vi "Alle Frontpanels auslesen.vi"(8 "Fehler (Eingang, kein Fehler)":errorcluster) -> (0 "Fehler (Ausgang)":errorcluster)   [LabVIEW 2020, in "Sprachverwaltung.lvlib"]
uses:
  Sprachverwaltung.lvlib
  Seiten/System Einstellungen V2/Aktioen FGV System Konstanten.ctl
  VI Anlagengrenzwerte.vi
  VI Gaszuordnung.vi
  VisBx Anzeige.vi
  Seiten/Grafik/VI Graph.vi
  Seiten/Grafik/Einstellungen Diagramme.vi
  VI Konfig FT-IR.vi
  Seiten/FT-IR/Gasliste vergleichen.vi
  Seiten/FT-IR/Algebraic Modul/VI Algebraic Konfig.vi
  Seiten/FT-IR/Get Spectra/get Spectra.vi
  VI Erw. Konfig.vi
  AK-Schnittstelle/Konfig AK.vi
  Seiten/Erweiterte Konfig/Status Steuerung.vi
  Seiten/Erweiterte Konfig/PID-Parameter Druckregler einstellen v2.vi
  Seiten/Erweiterte Konfig/Dichtheitstest.vi
  T90/T90 konfig.vi
  T90/T90 main.vi
  Seiten/FT-IR/Hintergrund durchfuehren.vi
  Seiten/System Einstellungen V2/System und Gaseinstellung V2.vi
  Seiten/Statusuebersicht/VI Statusuebersicht.vi
  Passwortverwaltung/VI Passwortverwaltung.vi
  Passwortverwaltung/Passwortlevel aendern.vi
  VI Anlagengrenzwerte PNS.vi
  PNS/Diagnose PNS.vi
  Allgemein/Runtime beenden.vi
  Allgemein/Bitte Warten.vi
  VI Stoermeldungen.vi
  VI Stoermeldepuffer.vi
  VI Stoermeldung Konfig.vi
  cRIO Ueberwachung/VI Fehlerliste.vi
  Seiten/Grafik/Kurven anzeigen.vi
  EPA 1065/Dichtheitstest 1065-345/Konfig Leak Check.vi
  Seiten/FT-IR/Konfig Recipes.vi
  Seiten/FT-IR/TOOLweb Interface Library/TOOLweb Rezept wechseln.vi
  Allgemein/Diagnose Zykluszeit.vi
  Linearisierung V2/SpanEinstellungen/show LIN Load Errors.vi
  EPA 1065/Interference verificaton 1065-366/Hilfe.vi
  EPA 1065/Interference verificaton 1065-375/VI Interference Konfig.vi
  Seiten/FT-IR/Span/Kalibrierung laden.vi
  VI Konfiguration Kalibriergase.vi
  EPA 1065/Interference verificaton 1065-366/VI Interference Konfig.vi
  Seiten/Erweiterte Konfig/Parameter Druck Sensoren.vi
  Seiten/EL3000/PMA/VI PMA Konfig.vi
  Seiten/EL3000/Allgemeine VI/Kalibrierdaten.vi
  Seiten/EL3000/FID/VI FID Konfig.vi
  Seiten/EL3000/Allgemeine VI/FID Manuell Kalibrieren.vi
  Seiten/EL3000/PMA/Kalibrieren/PMA Manuell Kalibrieren.vi
  Allgemein/SPRACHE.vi
  SysLog/VI SysLog History.vi
  SysLog/SysLog Status.vi
  Seiten/Erweiterte Konfig/Konfig CG-Check/CG-Test.vi
  Seiten/Erweiterte Konfig/Konfig CG-Check/VI CG-Check Konfig.vi
  Linearisierung V2/Gasteiler/Horiba/GDC Manuell.vi
  Backup mit WebDAV/Backup.vi
  Seiten/FT-IR/Span/VI Span Seite.vi
  Seiten/CalGas Aufschaltung/Aufschaltung_Popup.vi
  Auto Kalibrieren/VI Auto Kalibrieren.vi
  Linearisierung V2/VI Linearisierung v2.vi
  O2 Dichtheitstest/O2 main.vi
  Seiten/Erweiterte Konfig/Konfig CG-Check/CG_Auswertung.vi
  Linearisierung V2/Gasteiler/Gasteiler Korrektur.vi
  SprachEditor.vi
  EPA 1065/T90 1065-308/T90 Test Konfig.vi
  Schedule Modul/VI Schedule Seite.vi
  Linearisierung V2/Hintergrund durchfuehren FT-IR.vi
  EPA 1065/Gas Analyzer Drift 1065-550/Drift Verification Konfig.vi
  EPA 1065/HovaCAL Interference verification/VI Interference Konfig.vi
  Seiten/System Einstellungen V2/System Einstellungen V2.lvlib
  Seiten/Anlagengrenzwerte/Anlagengrenzwerte.lvlib
  Seiten/Gaszuordnung AO/Gaszuordnung AO.lvlib
  Seiten/Anlagenuebersicht/VisBx Anzeige/Anlagenuebersicht.lvlib
  Seiten/Grafik/Grafik.lvlib
  Seiten/FT-IR/FT-IR.lvlib
  Seiten/FT-IR/Algebraic Modul/Algebraic Modul.lvlib
  Seiten/FT-IR/Get Spectra/Get Spectra.lvlib
  Seiten/Erweiterte Konfig/Erweiterte Konfig.lvlib
  AK-Schnittstelle/AK-Schnittstelle.lvlib
  T90/T90.lvlib
  Seiten/Statusuebersicht/Statusuebersicht.lvlib
  Passwortverwaltung/Passwort.lvlib
  PNS/PNS.lvlib
  Allgemein/allgemeine Sub-VIs.lvlib
  Stoerungen/Stoerungen.lvlib
  cRIO Ueberwachung/cRIO Ueberwachung.lvlib
  EPA 1065/Dichtheitstest 1065-345/Dichtheitstest 1065-345.lvlib
  Seiten/FT-IR/TOOLweb Interface Library/TOOLweb Interface.lvlib
  Seiten/CalGas Aufschaltung/CalGas Aufschaltung.lvlib
  EPA 1065/Interference verificaton 1065-366/Interference verificaton 1065-366.lvlib
  Seiten/EL3000/PMA/PMA.lvlib
  Seiten/EL3000/FID/FID.lvlib
  Seiten/EL3000/Allgemeine VI/Allgemeine VI.lvlib
  Seiten/EL3000/PMA/Kalibrieren/Kalibrieren.lvlib
  SysLog/SysLog.lvlib
  Backup mit WebDAV/Backup.lvlib
  Seiten/FT-IR/Span/Spanfaktor.lvlib
  Seiten/Erweiterte Konfig/Konfig CG-Check/CG-Check Konfig.lvlib
  Auto Kalibrieren/Auto Kalibrieren.lvlib
  Linearisierung V2/Linearisierung v2.lvlib
  O2 Dichtheitstest/O2 Dichtheitstest.lvlib
  Linearisierung V2/Gasteiler/Horiba/Horiba GDC.lvlib
  Linearisierung V2/Gasteiler/Gasteiler.lvlib
  EPA 1065/T90 1065-308/T90 Test 1065-308.lvlib
  EPA 1065/ANR Test 1065-305/ARN Test 1065-305.lvlib
  EPA 1065/Interference verificaton 1065-375/Interference verificaton 1065-375.lvlib
  Schedule Modul/Schedule Modul.lvlib
  Seiten/Log Konfig/LogKonfig.lvlib
  EPA 1065/Gas Analyzer Drift 1065-550/Gas Analyzer Drift 1065-550.lvlib
  EPA 1065/Interference verificaton 1065-375/PDF_Interface_PDF Protokoll EPA1065_InterferenceVerification.vi
  EPA 1065/Interference verificaton 1065-366/PDF_Interface_PDF Protokoll EPA1065_InterferenceVerification.vi
  EPA 1065/ANR Test 1065-305/PDF_Interface_PDF Protokoll EPA1065_305 ARN.vi
  Linearisierung V2/Protokoll/PDF_Interface_PDF Protokoll EPA1065_307.vi
  Linearisierung V2/Protokoll/Protokoll.lvlib
  Linearisierung V2/Protokoll/PDF_Interface_PDF Protokoll Linearisierung.vi
  Seiten/Erweiterte Konfig/PDF_Interface_PDF Protokoll Dichtheitstest.vi
  O2 Dichtheitstest/PDF_Interface_PDF Protokoll O2 Leaktest.vi
  Hangup Check/PDF_Interface_PDF Protokoll HangUp.vi
  Hangup Check/Hangup Check.lvlib
  T90/PDF_Interface_PDF Protokoll T90.vi
  EPA 1065/T90 1065-308/PDF_Interface_PDF Protokoll EPA1065_308 T90.vi
  EPA 1065/Gas Analyzer Drift 1065-550/PDF_Interface_PDF Protokoll EPA1065_550 Drift.vi
  Linearisierung V2/SpanEinstellungen/SpanEinstellungen.lvlib
  EPA 1065/HovaCAL Interference verification/HovaCAL Interference verificaton.lvlib
panel:
  # "Durch ausführen des VI´s werden alle Frontpanels\ndie man vorher hinzufügt ausgelesen"
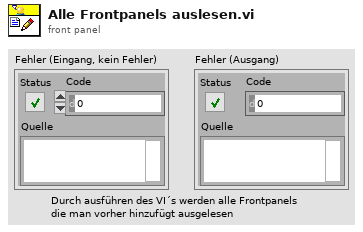
[diagram p1: front panel]
types:
  T1 = typedef "System Einstellungen V2.lvlib/Aktioen FGV System Konstanten.ctl" = enum16{"lesen", "laden", "speichern", "Sprache"}
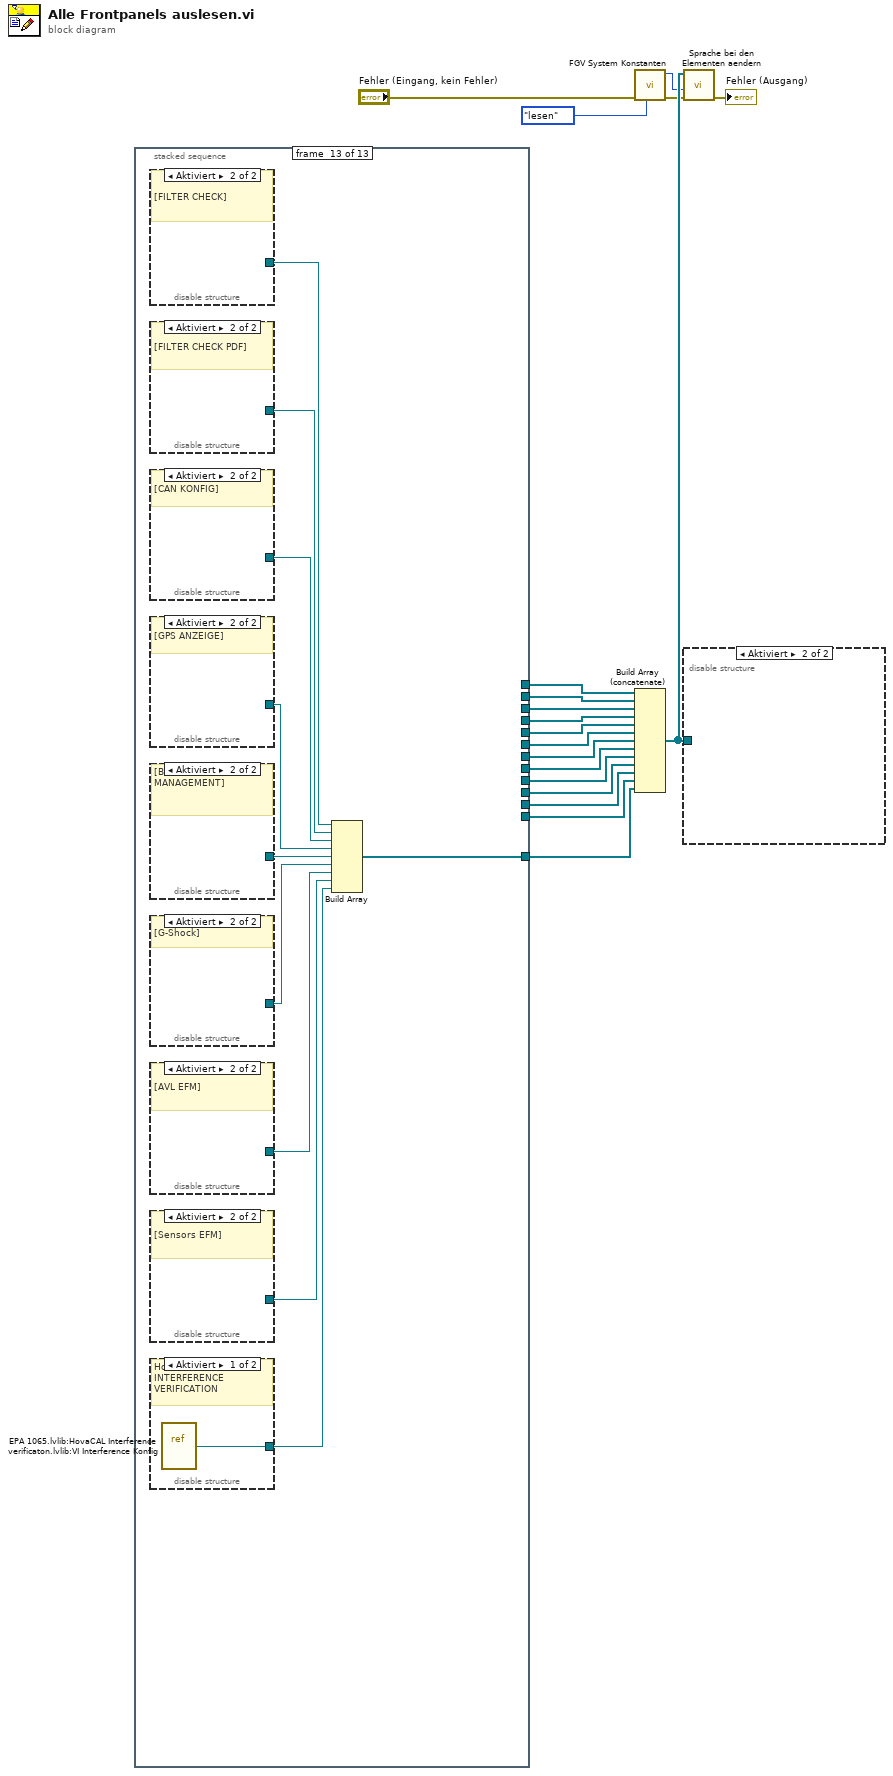
[diagram p0: block diagram]
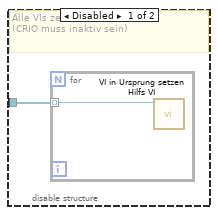
[diagram p2: hidden frame]
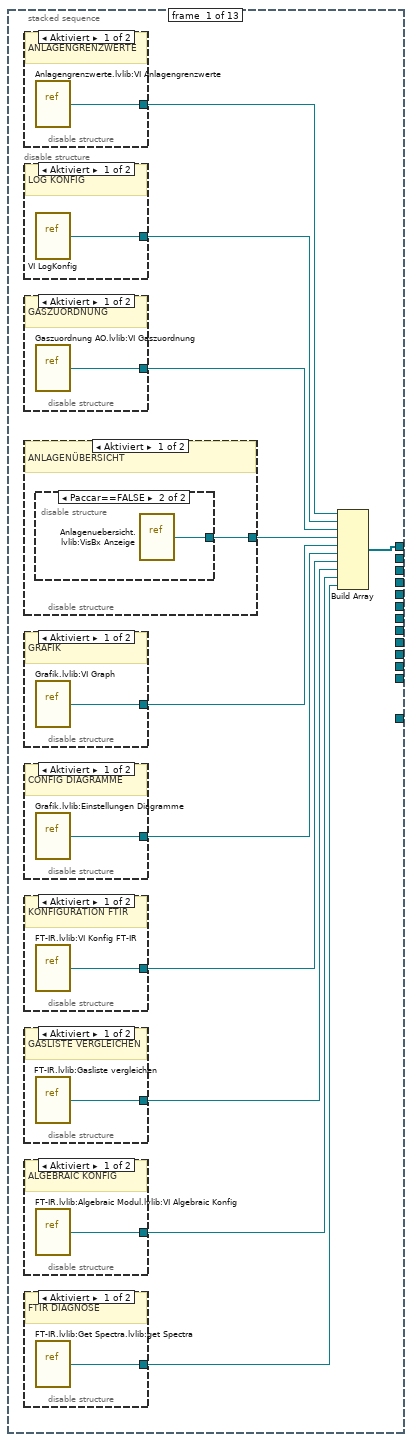
[diagram p3: hidden frame]
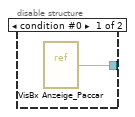
[diagram p10: hidden frame]
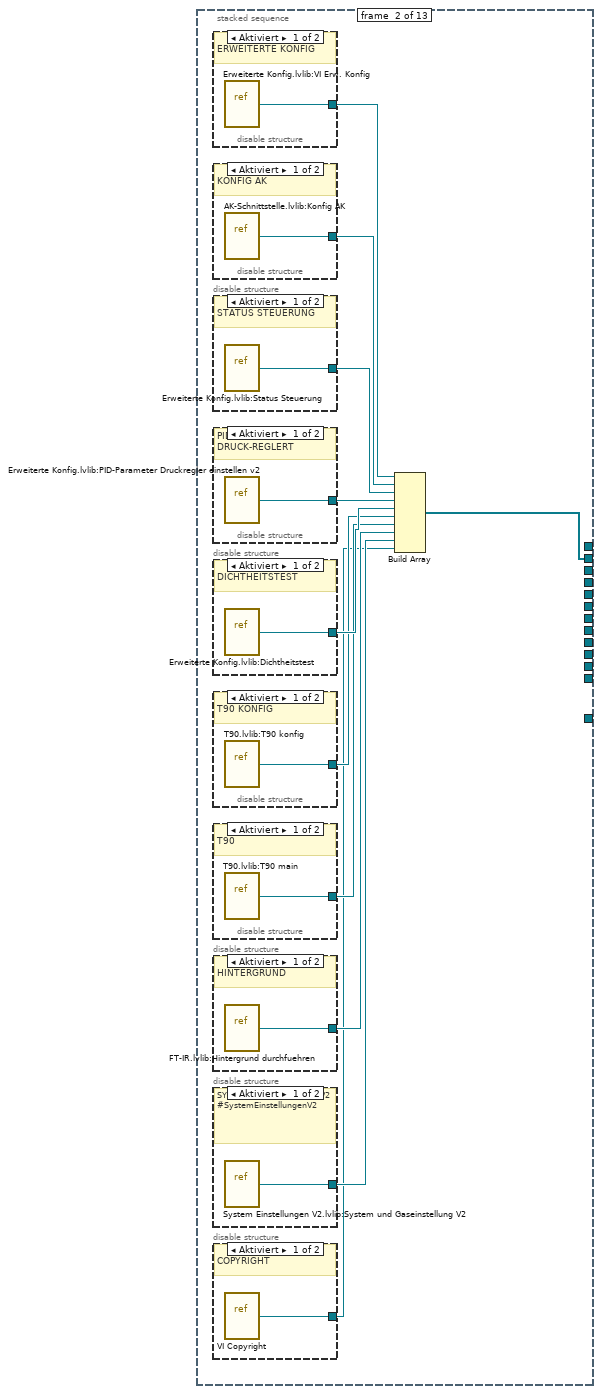
[diagram p15: hidden frame]
diagram:
  n1 = stacked-sequence {
    tunnel: [w20 _ _ _ _ _ _ _ _ _ _ _ _] -> w18
    tunnel: [_ w43 _ _ _ _ _ _ _ _ _ _ _] -> w17
    tunnel: [_ _ w64 _ _ _ _ _ _ _ _ _ _] -> w16
    tunnel: [_ _ _ w85 _ _ _ _ _ _ _ _ _] -> w15
    tunnel: [_ _ _ _ w109 _ _ _ _ _ _ _ _] -> w14
    tunnel: [_ _ _ _ _ w136 _ _ _ _ _ _ _] -> w13
    tunnel: [_ _ _ _ _ _ w151 _ _ _ _ _ _] -> w12
    tunnel: [_ _ _ _ _ _ _ w178 _ _ _ _ _] -> w11
    tunnel: [_ _ _ _ _ _ _ _ w199 _ _ _ _] -> w10
    tunnel: [_ _ _ _ _ _ _ _ _ w220 _ _ _] -> w9
    tunnel: [_ _ _ _ _ _ _ _ _ _ w234 _ _] -> w7
    tunnel: [_ _ _ _ _ _ _ _ _ _ _ w256 _] -> w2
    tunnel: [_ _ _ _ _ _ _ _ _ _ _ _ w278] -> w1
    frame #0 {
      n2 = disable-structure shown="Aktiviert" {
        disable-tunnel: [w42 _] -> w30
        frame Enabled {
          # "ANLAGENGRENZWERTE"
          n3 = vi-ref "Anlagengrenzwerte.lvlib:VI Anlagengrenzwerte.vi"() -> (w42:refnum<vi>)
        }
        frame Disabled {
        }
      }
      n4 = disable-structure shown="Aktiviert" {
        disable-tunnel: [w41 _] -> w29
        frame Enabled {
          # "LOG KONFIG"
          n5 = vi-ref "VI LogKonfig.vi"() -> (w41:refnum<vi>)
        }
        frame Disabled {
        }
      }
      n6 = disable-structure shown="Aktiviert" {
        disable-tunnel: [w40 _] -> w28
        frame Enabled {
          # "GASZUORDNUNG"
          n7 = vi-ref "Gaszuordnung AO.lvlib:VI Gaszuordnung.vi"() -> (w40:refnum<vi>)
        }
        frame Disabled {
        }
      }
      n8 = disable-structure shown="Aktiviert" {
        disable-tunnel: [w37 _] -> w27
        frame Enabled {
          # "ANLAGENÜBERSICHT"
          n9 = disable-structure shown="Paccar==FALSE" {
            disable-tunnel: [w38 w39] -> w37
            frame condition #0 {
              n10 = vi-ref "VisBx Anzeige_Paccar.vi"() -> (w38:refnum<vi>)
            }
            frame condition #1 (active) {
              n11 = vi-ref "Anlagenuebersicht.lvlib:VisBx Anzeige.vi"() -> (w39:refnum<vi>)
            }
          }
        }
        frame Disabled {
        }
      }
      n12 = disable-structure shown="Aktiviert" {
        disable-tunnel: [w36 _] -> w26
        frame Enabled {
          # "GRAFIK"
          n13 = vi-ref "Grafik.lvlib:VI Graph.vi"() -> (w36:refnum<vi>)
        }
        frame Disabled {
        }
      }
      n14 = disable-structure shown="Aktiviert" {
        disable-tunnel: [w35 _] -> w25
        frame Enabled {
          # "CONFIG DIAGRAMME"
          n15 = vi-ref "Grafik.lvlib:Einstellungen Diagramme.vi"() -> (w35:refnum<vi>)
        }
        frame Disabled {
        }
      }
      n16 = disable-structure shown="Aktiviert" {
        disable-tunnel: [w34 _] -> w24
        frame Enabled {
          # "KONFIGURATION FTIR"
          n17 = vi-ref "FT-IR.lvlib:VI Konfig FT-IR.vi"() -> (w34:refnum<vi>)
        }
        frame Disabled {
        }
      }
      n18 = disable-structure shown="Aktiviert" {
        disable-tunnel: [w33 _] -> w23
        frame Enabled {
          # "GASLISTE VERGLEICHEN"
          n19 = vi-ref "FT-IR.lvlib:Gasliste vergleichen.vi"() -> (w33:refnum<vi>)
        }
        frame Disabled {
        }
      }
      n20 = disable-structure shown="Aktiviert" {
        disable-tunnel: [w32 _] -> w22
        frame Enabled {
          # "ALGEBRAIC KONFIG"
          n21 = vi-ref "FT-IR.lvlib:Algebraic Modul.lvlib:VI Algebraic Konfig.vi"() -> (w32:refnum<vi>)
        }
        frame Disabled {
        }
      }
      n22 = disable-structure shown="Aktiviert" {
        disable-tunnel: [w31 _] -> w21
        frame Enabled {
          # "FTIR DIAGNOSE"
          n23 = vi-ref "FT-IR.lvlib:Get Spectra.lvlib:get Spectra.vi"() -> (w31:refnum<vi>)
        }
        frame Disabled {
        }
      }
      n24 = Build Array(w30, w29, w28, w27, w26, w25, w24, w23, w22, w21) -> (w20:refnum<vi>[])
    }
    frame #1 {
      n25 = disable-structure shown="Aktiviert" {
        disable-tunnel: [w63 _] -> w53
        frame Enabled {
          # "ERWEITERTE KONFIG"
          n26 = vi-ref "Erweiterte Konfig.lvlib:VI Erw. Konfig.vi"() -> (w63:refnum<vi>)
        }
        frame Disabled {
        }
      }
      n27 = disable-structure shown="Aktiviert" {
        disable-tunnel: [w62 _] -> w52
        frame Enabled {
          # "KONFIG AK"
          n28 = vi-ref "AK-Schnittstelle.lvlib:Konfig AK.vi"() -> (w62:refnum<vi>)
        }
        frame Disabled {
        }
      }
      n29 = disable-structure shown="Aktiviert" {
        disable-tunnel: [w61 _] -> w51
        frame Enabled {
          # "STATUS STEUERUNG"
          n30 = vi-ref "Erweiterte Konfig.lvlib:Status Steuerung.vi"() -> (w61:refnum<vi>)
        }
        frame Disabled {
        }
      }
      n31 = disable-structure shown="Aktiviert" {
        disable-tunnel: [w60 _] -> w50
        frame Enabled {
          # "PID PARAMETER DRUCK-REGLERT"
          n32 = vi-ref "Erweiterte Konfig.lvlib:PID-Parameter Druckregler einstellen v2.vi"() -> (w60:refnum<vi>)
        }
        frame Disabled {
        }
      }
      n33 = disable-structure shown="Aktiviert" {
        disable-tunnel: [w59 _] -> w49
        frame Enabled {
          # "DICHTHEITSTEST"
          n34 = vi-ref "Erweiterte Konfig.lvlib:Dichtheitstest.vi"() -> (w59:refnum<vi>)
        }
        frame Disabled {
        }
      }
      n35 = disable-structure shown="Aktiviert" {
        disable-tunnel: [w58 _] -> w48
        frame Enabled {
          # "T90 KONFIG"
          n36 = vi-ref "T90.lvlib:T90 konfig.vi"() -> (w58:refnum<vi>)
        }
        frame Disabled {
        }
      }
      n37 = disable-structure shown="Aktiviert" {
        disable-tunnel: [w57 _] -> w47
        frame Enabled {
          # "T90"
          n38 = vi-ref "T90.lvlib:T90 main.vi"() -> (w57:refnum<vi>)
        }
        frame Disabled {
        }
      }
      n39 = disable-structure shown="Aktiviert" {
        disable-tunnel: [w56 _] -> w46
        frame Enabled {
          # "HINTERGRUND"
          n40 = vi-ref "FT-IR.lvlib:Hintergrund durchfuehren.vi"() -> (w56:refnum<vi>)
        }
        frame Disabled {
        }
      }
      n41 = disable-structure shown="Aktiviert" {
        disable-tunnel: [w55 _] -> w45
        frame Enabled {
          # "SYSTEM EINSTELLUNGEN V2\n#SystemEinstellungenV2"
          n42 = vi-ref "System Einstellungen V2.lvlib:System und Gaseinstellung V2.vi"() -> (w55:refnum<vi>)
        }
        frame Disabled {
        }
      }
      n43 = disable-structure shown="Aktiviert" {
        disable-tunnel: [w54 _] -> w44
        frame Enabled {
          # "COPYRIGHT"
          n44 = vi-ref "VI Copyright.vi"() -> (w54:refnum<vi>)
        }
        frame Disabled {
        }
      }
      n45 = Build Array(w53, w52, w51, w50, w49, w48, w47, w46, w45, w44) -> (w43:refnum<vi>[])
    }
    frame #2 {
      n46 = disable-structure shown="Aktiviert" {
        disable-tunnel: [w84 _] -> w74
        frame Enabled {
          # "STATUSÜBERSICHT"
          n47 = vi-ref "Statusuebersicht.lvlib:VI Statusuebersicht.vi"() -> (w84:refnum<vi>)
        }
        frame Disabled {
        }
      }
      n48 = disable-structure shown="Aktiviert" {
        disable-tunnel: [w83 _] -> w73
        frame Enabled {
          # "PASSWORTVERWALTUNG"
          n49 = vi-ref "Passwort.lvlib:VI Passwortverwaltung.vi"() -> (w83:refnum<vi>)
        }
        frame Disabled {
        }
      }
      n50 = disable-structure shown="Aktiviert" {
        disable-tunnel: [w82 _] -> w72
        frame Enabled {
          # "PASSWORT AENDERN"
          n51 = vi-ref "Passwort.lvlib:Passwortlevel aendern.vi"() -> (w82:refnum<vi>)
        }
        frame Disabled {
        }
      }
      n52 = disable-structure shown="Aktiviert" {
        disable-tunnel: [w81 _] -> w71
        frame Enabled {
          # "FUNKTIONSTASTEN"
          n53 = vi-ref "VI Leer.vi"() -> (w81:refnum<vi>)
        }
        frame Disabled {
        }
      }
      n54 = disable-structure shown="Aktiviert" {
        disable-tunnel: [w80 _] -> w70
        frame Enabled {
          # "PNS"
          n55 = vi-ref "PNS.lvlib:VI Anlagengrenzwerte PNS.vi"() -> (w80:refnum<vi>)
        }
        frame Disabled {
        }
      }
      n56 = disable-structure shown="Aktiviert" {
        disable-tunnel: [w79 _] -> w69
        frame Enabled {
          # "DIAG PNS"
          n57 = vi-ref "PNS.lvlib:Diagnose PNS.vi"() -> (w79:refnum<vi>)
        }
        frame Disabled {
        }
      }
      n58 = disable-structure shown="Aktiviert" {
        disable-tunnel: [w78 _] -> w68
        frame Enabled {
          # "RUNTIME MENUE"
          n59 = vi-ref "VI Leer.vi"() -> (w78:refnum<vi>)
        }
        frame Disabled {
        }
      }
      n60 = disable-structure shown="Aktiviert" {
        disable-tunnel: [w77 _] -> w67
        frame Enabled {
          # "FAS06"
          n61 = vi-ref "Versa_06.vi"() -> (w77:refnum<vi>)
        }
        frame Disabled {
        }
      }
      n62 = disable-structure shown="Aktiviert" {
        disable-tunnel: [w76 _] -> w66
        frame Enabled {
          # "PERMANENT BEREICH"
          n63 = vi-ref "VI Permanent.vi"() -> (w76:refnum<vi>)
        }
        frame Disabled {
        }
      }
      n64 = disable-structure shown="Aktiviert" {
        disable-tunnel: [w75 _] -> w65
        frame Enabled {
          # "RUNTIME BEENDEN"
          n65 = vi-ref "allgemeine Sub-VIs.lvlib:Runtime beenden.vi"() -> (w75:refnum<vi>)
        }
        frame Disabled {
        }
      }
      n66 = Build Array(w74, w73, w72, w71, w70, w69, w68, w67, w66, w65) -> (w64:refnum<vi>[])
    }
    frame #3 {
      n67 = disable-structure shown="Aktiviert" {
        disable-tunnel: [w103 _] -> w95
        frame Enabled {
          # "SPEICHERN"
          n68 = vi-ref "allgemeine Sub-VIs.lvlib:Bitte Warten.vi"() -> (w103:refnum<vi>)
        }
        frame Disabled {
        }
      }
      n69 = disable-structure shown="Aktiviert" {
        disable-tunnel: [w102 _] -> w94
        frame Enabled {
          # "STOERMELDUNGEN"
          n70 = vi-ref "Stoerungen.lvlib:VI Stoermeldungen.vi"() -> (w102:refnum<vi>)
        }
        frame Disabled {
        }
      }
      n71 = disable-structure shown="Aktiviert" {
        disable-tunnel: [w101 _] -> w93
        frame Enabled {
          # "STOERMELDEPUFFER"
          n72 = vi-ref "Stoerungen.lvlib:VI Stoermeldepuffer.vi"() -> (w101:refnum<vi>)
        }
        frame Disabled {
        }
      }
      n73 = disable-structure shown="Aktiviert" {
        disable-tunnel: [w100 _] -> w92
        frame Enabled {
          # "STOERMELDE-KONFIG"
          n74 = vi-ref "Stoerungen.lvlib:VI Stoermeldung Konfig.vi"() -> (w100:refnum<vi>)
        }
        frame Disabled {
        }
      }
      n75 = disable-structure shown="Aktiviert" {
        disable-tunnel: [w99 _] -> w91
        frame Enabled {
          # "STOERMELDUNGSDATEI"
          n76 = vi-ref "VI Leer.vi"() -> (w99:refnum<vi>)
        }
        frame Disabled {
        }
      }
      n77 = disable-structure shown="Aktiviert" {
        disable-tunnel: [w98 _] -> w90
        frame Enabled {
          # "ERWEITERTE GASLISTE"
          n78 = vi-ref "VI Leer.vi"() -> (w98:refnum<vi>)
        }
        frame Disabled {
        }
      }
      n79 = disable-structure shown="Deaktiviert" {
        disable-tunnel: [w105 _] -> w89
        frame Disabled {
          # "LINEARISIERUNG FTIR"
          n80 = vi-ref "VI Leer.vi"() -> (w105:refnum<vi>)
        }
        frame Enabled {
        }
      }
      n81 = disable-structure shown="Aktiviert" {
        disable-tunnel: [w97 _] -> w88
        frame Enabled {
          # "ARN TEST"
          n82 = vi-ref "ARN Test Konfig v2.vi"() -> (w97:refnum<vi>)
        }
        frame Disabled {
        }
      }
      n83 = disable-structure shown="Aktiviert" {
        disable-tunnel: [w104 _] -> w87
        frame Disabled {
          # "ARN PROTOKOLL"
          n84 = vi-ref "EPA 1065.lvlib:ARN Test 1065-305.lvlib:PDF_Interface_PDF Protokoll EPA1065_305 ARN.vi"() -> (w104:refnum<vi>)
        }
        frame Enabled {
          # "PDF Interface"
        }
      }
      n85 = disable-structure shown="Aktiviert" {
        disable-tunnel: [w96 _] -> w86
        frame Enabled {
          # "FEHLER STEUERUNG"
          n86 = vi-ref "cRIO Ueberwachung.lvlib:VI Fehlerliste.vi"() -> (w96:refnum<vi>)
        }
        frame Disabled {
        }
      }
      n87 = Build Array(w95, w94, w93, w92, w91, w90, w89, w88, w87, w86) -> (w85:refnum<vi>[])
    }
    frame #4 {
      n88 = disable-structure shown="Deaktiviert" {
        disable-tunnel: [w119 _] -> w108
        frame Disabled {
          # "POLYNOMKOEFFIZIENTEN"
          n89 = vi-ref "VI Leer.vi"() -> (w119:refnum<vi>)
        }
        frame Enabled {
        }
      }
      n90 = disable-structure shown="Aktiviert" {
        disable-tunnel: [w118 _] -> w107
        frame Enabled {
          # "KONFIG LINEARITY VERIFICATION\n#Lin_Load_Err"
          n91 = vi-ref "Linearisierung v2.lvlib:SpanEinstellungen.lvlib:show LIN Load Errors.vi"() -> (w118:refnum<vi>)
        }
        frame Disabled {
        }
      }
      n92 = disable-structure shown="Deaktiviert" {
        disable-tunnel: [w117 _] -> w106
        frame Disabled {
          # "AUTO LIN VERIFICATION"
          n93 = vi-ref "VI Leer.vi"() -> (w117:refnum<vi>)
        }
        frame Enabled {
        }
      }
      n94 = disable-structure shown="Aktiviert" {
        disable-tunnel: [w126 _] -> w116
        frame Enabled {
          # "[GRAPHIK KURVEN]"
          n95 = vi-ref "Grafik.lvlib:Kurven anzeigen.vi"() -> (w126:refnum<vi>)
        }
        frame Disabled {
        }
      }
      n96 = disable-structure shown="Aktiviert" {
        disable-tunnel: [w123 _] -> w115
        frame Enabled {
          # "EPA DICHTHEITSTEST"
          n97 = vi-ref "EPA 1065.lvlib:Dichtheitstest 1065-345.lvlib:Konfig Leak Check.vi"() -> (w123:refnum<vi>)
        }
        frame Disabled {
        }
      }
      n98 = disable-structure shown="Aktiviert" {
        disable-tunnel: [w122 _] -> w114
        frame Enabled {
          # "REZEPT LADEN"
          n99 = vi-ref "FT-IR.lvlib:Konfig Recipes.vi"() -> (w122:refnum<vi>)
        }
        frame Disabled {
        }
      }
      n100 = disable-structure shown="Aktiviert" {
        disable-tunnel: [w121 _] -> w113
        frame Enabled {
          # "REZEPTWECHSEL"
          n101 = vi-ref "FT-IR.lvlib:TOOLweb Interface.lvlib:TOOLweb Rezept wechseln.vi"() -> (w121:refnum<vi>)
        }
        frame Disabled {
        }
      }
      n102 = disable-structure shown="Aktiviert" {
        disable-tunnel: [w120 _] -> w112
        frame Enabled {
          # "DIAG ZYKLUSZEIT"
          n103 = vi-ref "allgemeine Sub-VIs.lvlib:Diagnose Zykluszeit.vi"() -> (w120:refnum<vi>)
        }
        frame Disabled {
        }
      }
      n104 = disable-structure shown="Deaktiviert" {
        disable-tunnel: [w125 _] -> w111
        frame Disabled {
          # "EPA KONTROLLE PARAMETER"
          n105 = vi-ref "VI Leer.vi"() -> (w125:refnum<vi>)
        }
        frame Enabled {
        }
      }
      n106 = disable-structure shown="Deaktiviert" {
        disable-tunnel: [w124 _] -> w110
        frame Disabled {
          # "KONFIG GASTEILER"
          n107 = vi-ref "VI Leer.vi"() -> (w124:refnum<vi>)
        }
        frame Enabled {
        }
      }
      n108 = Build Array(w108, w107, w106, w116, w115, w114, w113, w112, w111, w110) -> (w109:refnum<vi>[])
    }
    frame #5 {
      n109 = disable-structure shown="Aktiviert" {
        disable-tunnel: [w142 _] -> w127
        frame Enabled {
          # "KALIBRIERDATEN LADEN"
          n110 = vi-ref "FT-IR.lvlib:Spanfaktor.lvlib:Kalibrierung laden.vi"() -> (w142:refnum<vi>)
        }
        frame Disabled {
        }
      }
      n111 = disable-structure shown="Aktiviert" {
        disable-tunnel: [refnum<vi> refnum ("vi reference") _] -> w128
        frame Enabled {
          # "KONTROLLE PARAMETER VOR LIN"
        }
        frame Disabled {
        }
      }
      n112 = disable-structure shown="Aktiviert" {
        disable-tunnel: [w141 _] -> w129
        frame Enabled {
          # "KONFIGURATION KALIBRIERGASE"
          n113 = vi-ref "CalGas Aufschaltung.lvlib:VI Konfiguration Kalibriergase.vi"() -> (w141:refnum<vi>)
        }
        frame Disabled {
        }
      }
      n114 = disable-structure shown="Aktiviert" {
        disable-tunnel: [w140 _] -> w130
        frame Enabled {
          # "INTERFERENCE VERIFICATION"
          n115 = vi-ref "EPA 1065.lvlib:Interference verificaton 1065-366.lvlib:VI Interference Konfig.vi"() -> (w140:refnum<vi>)
        }
        frame Disabled {
        }
      }
      n116 = disable-structure shown="Aktiviert" {
        disable-tunnel: [w144 _] -> w135
        frame Enabled {
          # "N2O Querempfindlichkeit"
          n117 = vi-ref "EPA 1065.lvlib:Interference verificaton 1065-375.lvlib:VI Interference Konfig.vi"() -> (w144:refnum<vi>)
        }
        frame Disabled {
        }
      }
      n118 = disable-structure shown="Deaktiviert" {
        disable-tunnel: [w145 _] -> w134
        frame Disabled {
          # "N2O Querempfindlichkeit"
          n119 = vi-ref "EPA 1065.lvlib:Interference verificaton 1065-375.lvlib:PDF_Interface_PDF Protokoll EPA1065_InterferenceVerification.vi"() -> (w145:refnum<vi>)
        }
        frame Enabled {
          # "PDF Interface"
        }
      }
      n120 = disable-structure shown="Deaktiviert" {
        disable-tunnel: [w139 _] -> w137
        frame Disabled {
          # "INTERFERENCE PROTOKOLL"
          n121 = vi-ref "EPA 1065.lvlib:Interference verificaton 1065-366.lvlib:PDF_Interface_PDF Protokoll EPA1065_InterferenceVerification.vi"() -> (w139:refnum<vi>)
        }
        frame Enabled {
          # "PDF Interface"
        }
      }
      n122 = disable-structure shown="Aktiviert" {
        disable-tunnel: [w146 _] -> w132
        frame Enabled {
          # "INTERFERENCE HILFE"
          n123 = vi-ref "EPA 1065.lvlib:Interference verificaton 1065-366.lvlib:Hilfe.vi"() -> (w146:refnum<vi>)
        }
        frame Disabled {
        }
      }
      n124 = disable-structure shown="Aktiviert" {
        disable-tunnel: [w138 _] -> w131
        frame Enabled {
          # "INTERFERENCE HILFE"
          n125 = vi-ref "EPA 1065.lvlib:Interference verificaton 1065-366.lvlib:Hilfe.vi"() -> (w138:refnum<vi>)
        }
        frame Disabled {
        }
      }
      n126 = disable-structure shown="Deaktiviert" {
        disable-tunnel: [w147 _] -> w133
        frame Disabled {
          # "SPUELEN"
          n127 = vi-ref "VI Leer.vi"() -> (w147:refnum<vi>)
        }
        frame Enabled {
        }
      }
      n128 = Build Array(w127, w128, w129, w130, w135, w134, w137, w132, w131, w133) -> (w136:refnum<vi>[])
    }
    frame #6 {
      n129 = disable-structure shown="Deaktiviert" {
        disable-tunnel: [w168 _] -> w158
        frame Disabled {
          # "Zu kopierender Case"
          # "GASTEILER KALIBRIEREN"
          n130 = vi-ref "VI Leer.vi"() -> (w168:refnum<vi>)
        }
        frame Enabled {
        }
      }
      n131 = disable-structure shown="Aktiviert" {
        disable-tunnel: [w167 _] -> w157
        frame Enabled {
          # "SENSOR KONFIGURATION"
          n132 = vi-ref "Erweiterte Konfig.lvlib:Parameter Druck Sensoren.vi"() -> (w167:refnum<vi>)
        }
        frame Disabled {
        }
      }
      n133 = disable-structure shown="Aktiviert" {
        disable-tunnel: [w166 _] -> w156
        frame Enabled {
          # "KONFIGURATION PMA"
          n134 = vi-ref "ABB-EL3000.lvlib:PMA.lvlib:VI PMA Konfig.vi"() -> (w166:refnum<vi>)
        }
        frame Disabled {
        }
      }
      n135 = disable-structure shown="Aktiviert" {
        disable-tunnel: [w165 _] -> w153
        frame Enabled {
          # "KALIBRIERDATEN"
          n136 = vi-ref "ABB-EL3000.lvlib:Allgemeine VI.lvlib:Kalibrierdaten.vi"() -> (w165:refnum<vi>)
        }
        frame Disabled {
        }
      }
      n137 = disable-structure shown="Aktiviert" {
        disable-tunnel: [w164 _] -> w152
        frame Enabled {
          # "KONFIGURATION FID"
          n138 = vi-ref "ABB-EL3000.lvlib:FID.lvlib:VI FID Konfig.vi"() -> (w164:refnum<vi>)
        }
        frame Disabled {
        }
      }
      n139 = disable-structure shown="Aktiviert" {
        disable-tunnel: [w163 _] -> w155
        frame Enabled {
          # "ABB MANUELL KALIBRIEREN"
          n140 = vi-ref "ABB-EL3000.lvlib:Allgemeine VI.lvlib:FID Manuell Kalibrieren.vi"() -> (w163:refnum<vi>)
        }
        frame Disabled {
        }
      }
      n141 = disable-structure shown="Aktiviert" {
        disable-tunnel: [w162 _] -> w154
        frame Enabled {
          # "PMA MANUELL KALIBRIEREN"
          n142 = vi-ref "ABB-EL3000.lvlib:PMA.lvlib:Kalibrieren.lvlib:PMA Manuell Kalibrieren.vi"() -> (w162:refnum<vi>)
        }
        frame Disabled {
        }
      }
      n143 = disable-structure shown="Aktiviert" {
        disable-tunnel: [w161 _] -> w150
        frame Enabled {
          # "SPRACHAUSWAHL"
          n144 = vi-ref "allgemeine Sub-VIs.lvlib:SPRACHE.vi"() -> (w161:refnum<vi>)
        }
        frame Disabled {
        }
      }
      n145 = disable-structure shown="Aktiviert" {
        disable-tunnel: [w160 _] -> w149
        frame Enabled {
          # "SYS LOG HISTORY"
          n146 = vi-ref "SysLog.lvlib:VI SysLog History.vi"() -> (w160:refnum<vi>)
        }
        frame Disabled {
        }
      }
      n147 = disable-structure shown="Aktiviert" {
        disable-tunnel: [w159 _] -> w148
        frame Enabled {
          # "SYS LOG STATUS"
          n148 = vi-ref "SysLog.lvlib:SysLog Status.vi"() -> (w159:refnum<vi>)
        }
        frame Disabled {
        }
      }
      n149 = Build Array(w158, w157, w156, w153, w152, w155, w154, w150, w149, w148) -> (w151:refnum<vi>[])
    }
    frame #7 {
      n150 = disable-structure shown="Aktiviert" {
        disable-tunnel: [w185 _] -> w179
        frame Enabled {
          # "PNS UEBERSICHT"
          n151 = vi-ref "PNS.lvlib:PNS Anlagenuebersicht.lvlib:VisBx Anzeige PNS.vi"() -> (w185:refnum<vi>)
        }
        frame Disabled {
        }
      }
      n152 = disable-structure shown="Aktiviert" {
        disable-tunnel: [w189 _] -> w177
        frame Enabled {
          # "CG TEST"
          n153 = vi-ref "Erweiterte Konfig.lvlib:CG-Check Konfig.lvlib:CG-Test.vi"() -> (w189:refnum<vi>)
        }
        frame Disabled {
        }
      }
      n154 = disable-structure shown="Aktiviert" {
        disable-tunnel: [w188 _] -> w176
        frame Enabled {
          # "KONFIG CG CHECK"
          n155 = vi-ref "Erweiterte Konfig.lvlib:CG-Check Konfig.lvlib:VI CG-Check Konfig.vi"() -> (w188:refnum<vi>)
        }
        frame Disabled {
        }
      }
      n156 = disable-structure shown="Deaktiviert" {
        disable-tunnel: [w187 _] -> w175
        frame Disabled {
          n157 = vi-ref "PNS.lvlib:PNS Anlagenuebersicht.lvlib:VisBx Anzeige PNS.vi"() -> (w187:refnum<vi>)
        }
        frame Enabled {
        }
      }
      n158 = disable-structure shown="Aktiviert" {
        disable-tunnel: [w186 _] -> w174
        frame Enabled {
          # "HORIBA GDC"
          n159 = vi-ref "Linearisierung v2.lvlib:Gasteiler.lvlib:Horiba GDC.lvlib:GDC Manuell.vi"() -> (w186:refnum<vi>)
        }
        frame Disabled {
        }
      }
      n160 = disable-structure shown="Aktiviert" {
        disable-tunnel: [w184 _] -> w173
        frame Enabled {
          # "BACKUP"
          n161 = vi-ref "Backup.lvlib:Backup.vi"() -> (w184:refnum<vi>)
        }
        frame Disabled {
        }
      }
      n162 = disable-structure shown="Aktiviert" {
        disable-tunnel: [w183 _] -> w172
        frame Enabled {
          # "SPAN FAKTOREN"
          n163 = vi-ref "FT-IR.lvlib:Spanfaktor.lvlib:VI Span Seite.vi"() -> (w183:refnum<vi>)
        }
        frame Disabled {
        }
      }
      n164 = disable-structure shown="Aktiviert" {
        disable-tunnel: [w182 _] -> w171
        frame Enabled {
          # "CG POPUP"
          n165 = vi-ref "CalGas Aufschaltung.lvlib:Aufschaltung_Popup.vi"() -> (w182:refnum<vi>)
        }
        frame Disabled {
        }
      }
      n166 = disable-structure shown="Aktiviert" {
        disable-tunnel: [w181 _] -> w170
        frame Enabled {
          # "AUTO CALIBRATION"
          n167 = vi-ref "Auto Kalibrieren.lvlib:VI Auto Kalibrieren.vi"() -> (w181:refnum<vi>)
        }
        frame Disabled {
        }
      }
      n168 = disable-structure shown="Aktiviert" {
        disable-tunnel: [w180 _] -> w169
        frame Enabled {
          # "LIN V2"
          n169 = vi-ref "Linearisierung v2.lvlib:VI Linearisierung v2.vi"() -> (w180:refnum<vi>)
        }
        frame Disabled {
        }
      }
      n170 = Build Array(w179, w177, w176, w175, w174, w173, w172, w171, w170, w169) -> (w178:refnum<vi>[])
    }
    frame #8 {
      n171 = disable-structure shown="Aktiviert" {
        disable-tunnel: [w210 _] -> w200
        frame Enabled {
          # "O2 LEAKTEST"
          n172 = vi-ref "O2 Dichtheitstest.lvlib:O2 main.vi"() -> (w210:refnum<vi>)
        }
        frame Disabled {
        }
      }
      n173 = disable-structure shown="Aktiviert" {
        disable-tunnel: [w209 _] -> w198
        frame Enabled {
          # "CG TEST RESULT"
          n174 = vi-ref "Erweiterte Konfig.lvlib:CG-Check Konfig.lvlib:CG_Auswertung.vi"() -> (w209:refnum<vi>)
        }
        frame Disabled {
        }
      }
      n175 = disable-structure shown="Aktiviert" {
        disable-tunnel: [w208 _] -> w197
        frame Enabled {
          # "GASTEILER ABWEICHUNG"
          n176 = vi-ref "Linearisierung v2.lvlib:Gasteiler.lvlib:Gasteiler Korrektur.vi"() -> (w208:refnum<vi>)
        }
        frame Disabled {
        }
      }
      n177 = disable-structure shown="Deaktiviert" {
        disable-tunnel: [w207 _] -> w196
        frame Disabled {
          # "EPA LIN CHECK PROTOKOLL"
          n178 = vi-ref "Linearisierung v2.lvlib:Protokoll.lvlib:PDF_Interface_PDF Protokoll EPA1065_307.vi"() -> (w207:refnum<vi>)
        }
        frame Enabled {
          # "PDF Intervase"
        }
      }
      n179 = disable-structure shown="Deaktiviert" {
        disable-tunnel: [w201 _] -> w190
        frame Disabled {
          # "LIN CHECK PROTOKOLL"
          n180 = vi-ref "Linearisierung v2.lvlib:Protokoll.lvlib:PDF_Interface_PDF Protokoll Linearisierung.vi"() -> (w201:refnum<vi>)
        }
        frame Enabled {
          # "PDF Interface"
        }
      }
      n181 = disable-structure shown="Deaktiviert" {
        disable-tunnel: [w206 _] -> w191
        frame Disabled {
          # "LEAK CHECK PROTOKOLL"
          n182 = vi-ref "Erweiterte Konfig.lvlib:PDF_Interface_PDF Protokoll Dichtheitstest.vi"() -> (w206:refnum<vi>)
        }
        frame Enabled {
          # "PDF Interface"
        }
      }
      n183 = disable-structure shown="Deaktiviert" {
        disable-tunnel: [w205 _] -> w195
        frame Disabled {
          # "O2 LEAK PROTOKOLL"
          n184 = vi-ref "O2 Dichtheitstest.lvlib:PDF_Interface_PDF Protokoll O2 Leaktest.vi"() -> (w205:refnum<vi>)
        }
        frame Enabled {
          # "PDF Interface"
        }
      }
      n185 = disable-structure shown="Deaktiviert" {
        disable-tunnel: [w204 _] -> w194
        frame Disabled {
          # "HANG UP PROTOKOLL"
          n186 = vi-ref "Hangup Check.lvlib:PDF_Interface_PDF Protokoll HangUp.vi"() -> (w204:refnum<vi>)
        }
        frame Enabled {
          # "PDF Interface"
        }
      }
      n187 = disable-structure shown="Aktiviert" {
        disable-tunnel: [w203 _] -> w193
        frame Disabled {
          # "T90 PROTOKOLL"
          n188 = vi-ref "T90.lvlib:PDF_Interface_PDF Protokoll T90.vi"() -> (w203:refnum<vi>)
        }
        frame Enabled {
          # "PDF Interface"
        }
      }
      n189 = disable-structure shown="Aktiviert" {
        disable-tunnel: [w202 _] -> w192
        frame Enabled {
          # "SRACHEDITOR"
          n190 = vi-ref "Sprachverwaltung.lvlib:SprachEditor.vi"() -> (w202:refnum<vi>)
        }
        frame Disabled {
        }
      }
      n191 = Build Array(w200, w198, w197, w196, w190, w191, w195, w194, w193, w192) -> (w199:refnum<vi>[])
    }
    frame #9 {
      n192 = disable-structure shown="Aktiviert" {
        disable-tunnel: [w232 _] -> w221
        frame Disabled {
          # "SYSLOG MESSAGES"
          n193 = vi-ref "VI Leer.vi"() -> (w232:refnum<vi>)
        }
        frame Enabled {
          # "SYSLOG MESSAGES\n#SysLogCodes \ncRio"
        }
      }
      n194 = disable-structure shown="Aktiviert" {
        disable-tunnel: [w231 _] -> w219
        frame Disabled {
          # "SYSLOG MESSAGES"
          n195 = vi-ref "VI Leer.vi"() -> (w231:refnum<vi>)
        }
        frame Enabled {
          # "SYSLOG MESSAGES\n#SysLogCodes\nPC"
        }
      }
      n196 = disable-structure shown="Aktiviert" {
        disable-tunnel: [w227 _] -> w218
        frame Disabled {
          # "SYSLOG MESSAGES"
          n197 = vi-ref "VI Leer.vi"() -> (w227:refnum<vi>)
        }
        frame Enabled {
          # "SYSLOG MESSAGES\n#SysLogCodes\nPC"
        }
      }
      n198 = disable-structure shown="Aktiviert" {
        disable-tunnel: [w230 _] -> w217
        frame Enabled {
          # "T90 EPA\nTest"
          n199 = vi-ref "EPA 1065.lvlib:T90 Test 1065-308.lvlib:T90 Test Konfig.vi"() -> (w230:refnum<vi>)
        }
        frame Disabled {
          # "T90 EPA\nTest"
        }
      }
      n200 = disable-structure shown="Aktiviert" {
        disable-tunnel: [w229 _] -> w216
        frame Disabled {
          # "T90 EPA\nTest"
          n201 = vi-ref "EPA 1065.lvlib:T90 Test 1065-308.lvlib:PDF_Interface_PDF Protokoll EPA1065_308 T90.vi"() -> (w229:refnum<vi>)
        }
        frame Enabled {
          # "T90 EPA\nTest\nPDF Interface"
        }
      }
      n202 = disable-structure shown="Aktiviert" {
        disable-tunnel: [w228 _] -> w215
        frame Enabled {
          # "Scheduler"
          n203 = vi-ref "Schedule Modul.lvlib:VI Schedule Seite.vi"() -> (w228:refnum<vi>)
        }
        frame Disabled {
          # "Scheduler"
        }
      }
      n204 = disable-structure shown="Aktiviert" {
        disable-tunnel: [w226 _] -> w214
        frame Enabled {
          # "Hintergrund V2"
          n205 = vi-ref "Linearisierung v2.lvlib:Hintergrund durchfuehren FT-IR.vi"() -> (w226:refnum<vi>)
        }
        frame Disabled {
          # "Hintergrund V2"
        }
      }
      n206 = disable-structure shown="Aktiviert" {
        disable-tunnel: [w224 w225] -> w213
        frame Enabled {
          # "PDF Interface"
          n207 = vi-ref "VI Leer.vi"() -> (w224:refnum<vi>)
        }
        frame Disabled {
          # "[CG TEST PDF]\n#BugFix75"
          n208 = vi-ref "PDF_Interface_PDF Protokoll CalGas.vi"() -> (w225:refnum<vi>)
        }
      }
      n209 = disable-structure shown="Aktiviert" {
        disable-tunnel: [w223 _] -> w212
        frame Disabled {
          n210 = vi-ref "VI Leer.vi"() -> (w223:refnum<vi>)
        }
        frame Enabled {
          # "[CHILLER EPA TEST]"
        }
      }
      n211 = disable-structure shown="Aktiviert" {
        disable-tunnel: [w222 _] -> w211
        frame Disabled {
          n212 = vi-ref "VI Leer.vi"() -> (w222:refnum<vi>)
        }
        frame Enabled {
          # "[CHILLER EPA PROTOKOLL]"
        }
      }
      n213 = Build Array(w221, w219, w218, w217, w216, w215, w214, w213, w212, w211) -> (w220:refnum<vi>[])
    }
    frame #10 {
      n214 = disable-structure shown="Deaktiviert" {
        disable-tunnel: [w255 _] -> w243
        frame Disabled {
          # "SYSLOG MESSAGES"
          n215 = vi-ref "VI Leer.vi"() -> (w255:refnum<vi>)
        }
        frame Enabled {
          # "[FID O2 EPA TEST]"
        }
      }
      n216 = disable-structure shown="Aktiviert" {
        disable-tunnel: [w254 _] -> w242
        frame Disabled {
          # "SYSLOG MESSAGES"
          n217 = vi-ref "VI Leer.vi"() -> (w254:refnum<vi>)
        }
        frame Enabled {
          # "[FID O2 EPA PROTOKOLL]"
        }
      }
      n218 = disable-structure shown="Aktiviert" {
        disable-tunnel: [w252 w253] -> w241
        frame Disabled {
          # "SYSLOG MESSAGES"
          n219 = vi-ref "VI Leer.vi"() -> (w252:refnum<vi>)
        }
        frame Enabled {
          # "[DRIFT EPA TEST]"
          n220 = vi-ref "EPA 1065.lvlib:Gas Analyzer Drift 1065-550.lvlib:Drift Verification Konfig.vi"() -> (w253:refnum<vi>)
        }
      }
      n221 = disable-structure shown="Aktiviert" {
        disable-tunnel: [w248 w249] -> w238
        frame Enabled {
          # "PDF Interface"
          n222 = vi-ref "VI Leer.vi"() -> (w248:refnum<vi>)
        }
        frame Disabled {
          # "[DRIFT EPA PROTOKOLL]"
          n223 = vi-ref "EPA 1065.lvlib:Gas Analyzer Drift 1065-550.lvlib:PDF_Interface_PDF Protokoll EPA1065_550 Drift.vi"() -> (w249:refnum<vi>)
        }
      }
      n224 = disable-structure shown="Aktiviert" {
        disable-tunnel: [w247 _] -> w237
        frame Disabled {
          # "SYSLOG MESSAGES"
          n225 = vi-ref "VI Leer.vi"() -> (w247:refnum<vi>)
        }
        frame Enabled {
          # "[PRE EPA TEST]"
        }
      }
      n226 = disable-structure shown="Aktiviert" {
        disable-tunnel: [w246 _] -> w236
        frame Disabled {
          # "SYSLOG MESSAGES"
          n227 = vi-ref "VI Leer.vi"() -> (w246:refnum<vi>)
        }
        frame Enabled {
          # "[PRE EPA PROTOKOLL]"
        }
      }
      n228 = disable-structure shown="Aktiviert" {
        disable-tunnel: [w245 _] -> w235
        frame Disabled {
          # "SYSLOG MESSAGES"
          n229 = vi-ref "VI Leer.vi"() -> (w245:refnum<vi>)
        }
        frame Enabled {
          # "[FID OPTIMIZATION]"
        }
      }
      n230 = disable-structure shown="Aktiviert" {
        disable-tunnel: [w251 _] -> w240
        frame Disabled {
          n231 = vi-ref "VI Leer.vi"() -> (w251:refnum<vi>)
        }
        frame Enabled {
          # "[FID OPTIMIZATION PDF]"
        }
      }
      n232 = disable-structure shown="Aktiviert" {
        disable-tunnel: [w250 _] -> w239
        frame Disabled {
          n233 = vi-ref "VI Leer.vi"() -> (w250:refnum<vi>)
        }
        frame Enabled {
          # "[FID RESPONSE FAKTOR]"
        }
      }
      n234 = disable-structure shown="Aktiviert" {
        disable-tunnel: [w244 _] -> w233
        frame Disabled {
          n235 = vi-ref "VI Leer.vi"() -> (w244:refnum<vi>)
        }
        frame Enabled {
          # "[KONFIG ZIRCONIA]"
        }
      }
      n236 = Build Array(w243, w242, w241, w238, w237, w236, w235, w240, w239, w233) -> (w234:refnum<vi>[])
    }
    frame #11 {
      n237 = disable-structure shown="Aktiviert" {
        disable-tunnel: [w276 _] -> w266
        frame Disabled {
          n238 = vi-ref "VI Leer.vi"() -> (w276:refnum<vi>)
        }
        frame Enabled {
          # "[ZIRCONIA MANUELL KALIBRIEREN]"
        }
      }
      n239 = disable-structure shown="Aktiviert" {
        disable-tunnel: [w275 _] -> w265
        frame Disabled {
          n240 = vi-ref "VI Leer.vi"() -> (w275:refnum<vi>)
        }
        frame Enabled {
          # "[ARN EU PDF]"
        }
      }
      n241 = disable-structure shown="Aktiviert" {
        disable-tunnel: [w274 _] -> w264
        frame Disabled {
          n242 = vi-ref "VI Leer.vi"() -> (w274:refnum<vi>)
        }
        frame Enabled {
          # "[LEAK CHECK EU PDF]"
        }
      }
      n243 = disable-structure shown="Aktiviert" {
        disable-tunnel: [w271 _] -> w261
        frame Disabled {
          n244 = vi-ref "VI Leer.vi"() -> (w271:refnum<vi>)
        }
        frame Enabled {
          # "[T90 EU PDF]"
        }
      }
      n245 = disable-structure shown="Aktiviert" {
        disable-tunnel: [w270 _] -> w260
        frame Disabled {
          n246 = vi-ref "VI Leer.vi"() -> (w270:refnum<vi>)
        }
        frame Enabled {
          # "[LIN EU PDF]"
        }
      }
      n247 = disable-structure shown="Aktiviert" {
        disable-tunnel: [w269 _] -> w259
        frame Disabled {
          n248 = vi-ref "VI Leer.vi"() -> (w269:refnum<vi>)
        }
        frame Enabled {
          # "[NH3 DRIFT EU TEST]"
        }
      }
      n249 = disable-structure shown="Aktiviert" {
        disable-tunnel: [w268 _] -> w258
        frame Disabled {
          n250 = vi-ref "VI Leer.vi"() -> (w268:refnum<vi>)
        }
        frame Enabled {
          # "[NH3 DRIFT PDF]"
        }
      }
      n251 = disable-structure shown="Aktiviert" {
        disable-tunnel: [w273 _] -> w263
        frame Disabled {
          n252 = vi-ref "VI Leer.vi"() -> (w273:refnum<vi>)
        }
        frame Enabled {
          # "[NH3 INTERFERENCE PDF]"
        }
      }
      n253 = disable-structure shown="Aktiviert" {
        disable-tunnel: [w272 _] -> w262
        frame Disabled {
          n254 = vi-ref "VI Leer.vi"() -> (w272:refnum<vi>)
        }
        frame Enabled {
          # "[NH3 INTERFERENCE VERIFICATION]"
        }
      }
      n255 = disable-structure shown="Aktiviert" {
        disable-tunnel: [_ w267] -> w257
        frame Enabled {
          # "[CO2 INTERFERENCE VERIFICATION]"
        }
        frame Disabled {
          n256 = vi-ref "VI Leer.vi"() -> (w267:refnum<vi>)
        }
      }
      n257 = Build Array(w266, w265, w264, w261, w260, w259, w258, w263, w262, w257) -> (w256:refnum<vi>[])
    }
    frame #12 {
      n258 = disable-structure shown="Aktiviert" {
        disable-tunnel: [w295 _] -> w286
        frame Disabled {
          n259 = vi-ref "VI Leer.vi"() -> (w295:refnum<vi>)
        }
        frame Enabled {
          # "[FILTER CHECK]"
        }
      }
      n260 = disable-structure shown="Aktiviert" {
        disable-tunnel: [w294 _] -> w285
        frame Disabled {
          n261 = vi-ref "VI Leer.vi"() -> (w294:refnum<vi>)
        }
        frame Enabled {
          # "[FILTER CHECK PDF]"
        }
      }
      n262 = disable-structure shown="Aktiviert" {
        disable-tunnel: [w287 _] -> w277
        frame Disabled {
          n263 = vi-ref "VI Leer.vi"() -> (w287:refnum<vi>)
        }
        frame Enabled {
          # "[CAN KONFIG]"
        }
      }
      n264 = disable-structure shown="Aktiviert" {
        disable-tunnel: [w293 _] -> w284
        frame Disabled {
          n265 = vi-ref "VI Leer.vi"() -> (w293:refnum<vi>)
        }
        frame Enabled {
          # "[GPS ANZEIGE]"
        }
      }
      n266 = disable-structure shown="Aktiviert" {
        disable-tunnel: [w292 _] -> w283
        frame Disabled {
          n267 = vi-ref "VI Leer.vi"() -> (w292:refnum<vi>)
        }
        frame Enabled {
          # "[BATTERY MANAGEMENT]"
        }
      }
      n268 = disable-structure shown="Aktiviert" {
        disable-tunnel: [w291 _] -> w282
        frame Disabled {
          n269 = vi-ref "VI Leer.vi"() -> (w291:refnum<vi>)
        }
        frame Enabled {
          # "[G-Shock]"
        }
      }
      n270 = disable-structure shown="Aktiviert" {
        disable-tunnel: [w290 _] -> w281
        frame Disabled {
          n271 = vi-ref "VI Leer.vi"() -> (w290:refnum<vi>)
        }
        frame Enabled {
          # "[AVL EFM]"
        }
      }
      n272 = disable-structure shown="Aktiviert" {
        disable-tunnel: [w289 _] -> w280
        frame Disabled {
          n273 = vi-ref "VI Leer.vi"() -> (w289:refnum<vi>)
        }
        frame Enabled {
          # "[Sensors EFM]"
        }
      }
      n274 = disable-structure shown="Aktiviert" {
        disable-tunnel: [w288 _] -> w279
        frame Enabled {
          # "HovaCAL\nINTERFERENCE VERIFICATION"
          n275 = vi-ref "EPA 1065.lvlib:HovaCAL Interference verificaton.lvlib:VI Interference Konfig.vi"() -> (w288:refnum<vi>)
        }
        frame Disabled {
        }
      }
      n276 = Build Array(w286, w285, w277, w284, w283, w282, w281, w280, w279) -> (w278:refnum<vi>[])
    }
  }
  n277 = call "FGV System Konstanten.vi"("Aktionen"=Aktioen_FGV_System_Konstanten."lesen", "error in"="Fehler (Eingang, kein Fehler)") -> ("error out"=w6:errorcluster, "Sprachindex"=w3:u16)  [unwired: 5 in, 3 out]
  n278 = Build Array (concatenate)(w18, w17, w16, w15, w14, w13, w12, w11, w10, w9, w7, w2, w1) -> (w8:refnum<vi>[])
  n279 = call "Sprache bei den Elementen aendern.vi"("Fehler (Eingang, kein Fehler)"=w6, "Sprachauswahl"=w3, "VI Referenzen"=w8) -> ("Fehler (Ausgang)"=→"Fehler (Ausgang)":errorcluster)  [unwired: 7 in, 1 out]
  n280 = disable-structure shown="Aktiviert" {
    disable-tunnel: w8 -> [w296 _]
    frame Disabled {
      # "Alle VIs zentrieren\n(CRIO muss inaktiv sein)"
      n281 = for {
        tunnel: w296 -> [w297] mode=indexing
        n282 = call "VI in Ursprung setzen Hilfs VI.vi"("VI Referenz"=w297) -> ()  [unwired: 11 in]
      }
    }
    frame Enabled {
    }
  }
